vi "Email_transfer_global.vi"() -> ()   [LabVIEW 2020]
panel:
  in  "Started sending":timestamp
  in  "Busy?":bool
  in  "attachments":path[](array[path])
  in  "message":string
  in  "subject ([No Subject])":string="[No Subject]"
  in  "recipients":string[](array[string])
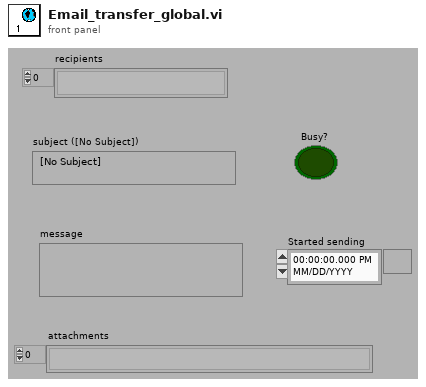
[diagram p1: front panel]
diagram:
